vi "Example 1.vi"(8 "error in (no error)":errorcluster) -> (0 "error out":errorcluster)   [LabVIEW 2021, in "Named Timers.lvlib"]
uses:
  Named Timers.lvlib
  bc7bc3af-0b1d-4bbd-b21e-fb7784355964.vi
  7345f343-11d4-4018-b647-47a13be3ef10.vi
  f1f7e482-33cc-452b-8412-1830cebe123d.vi
panel:
  out "Number of timers":i32
  out "Timers":string[](array[string])
  in  "Use case":enum16{"Use case 1", "Use case 2", "Use case 3"}(ring)
  out "Timer 3 Elapsed time (ms)":u32
  out "Timer 2 Elapsed time (ms)":u32
  out "Timer 1 Elapsed time (ms)":u32
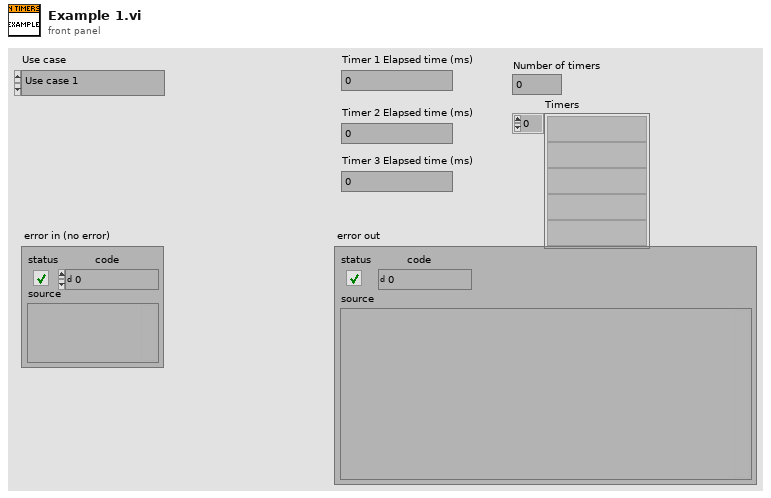
[diagram p1: front panel]
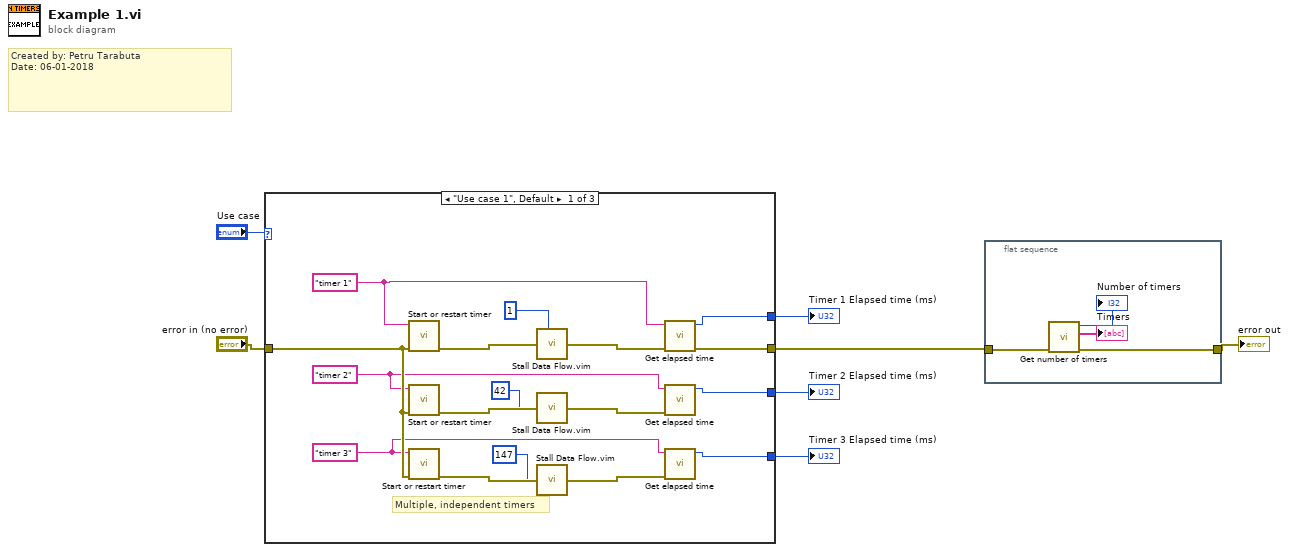
[diagram p0: block diagram]
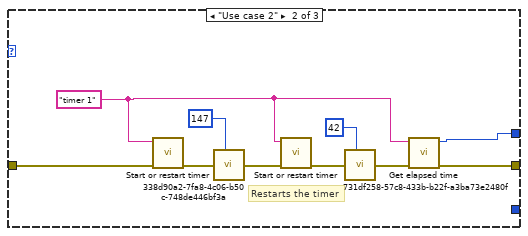
[diagram p2: hidden frame]
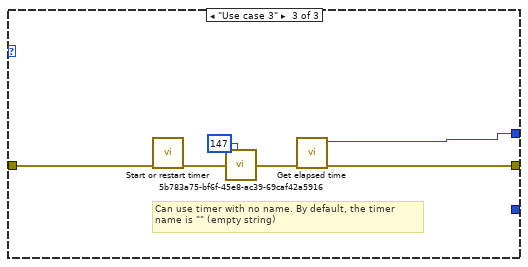
[diagram p3: hidden frame]
diagram:
  # "Created by: Petru Tarabuta\nDate: 06-01-2018"
  n1 = case shown="\"Use case 1\", Default" "Use case" {
    tunnel: [w24 w34 w40] -> w7
    tunnel: "error in (no error)" -> [w21 w31 w37]
    tunnel: [w10 _ _] -> w3
    tunnel: [w9 _ _] -> w2
    tunnel: [w8 w25 w35] -> w1
    frame "Use case 1", Default {
      w15 = "timer 3" ("Timer name")
      w19 = "timer 2" ("Timer name")
      w11 = "timer 1" ("Timer name")
      # "Multiple, independent timers"
      n2 = call "Start or restart timer.vi"("error in (no error)"=w21, "Timer name"=w11) -> ("error out"=w20:errorcluster)  [unwired: 9 in]
      n3 = call "Start or restart timer.vi"("error in (no error)"=w21, "Timer name"=w19) -> ("error out"=w18:errorcluster)  [unwired: 9 in]
      n4 = call "Start or restart timer.vi"("error in (no error)"=w21, "Timer name"=w15) -> ("error out"=w14:errorcluster)  [unwired: 9 in]
      n5 = call "Stall Data Flow.vim"("value in"=w20, "milliseconds to wait"=u32 1) -> ("value out"=w23:errorcluster)  [unwired: 1 out]
      n6 = call "Stall Data Flow.vim"("value in"=w18, "milliseconds to wait"=u32 42) -> ("value out"=w17:errorcluster)  [unwired: 1 out]
      n7 = call "Stall Data Flow.vim"("value in"=w14, "milliseconds to wait"=u32 147) -> ("value out"=w13:errorcluster)  [unwired: 1 out]
      n8 = call "Get elapsed time.vi"("error in (no error)"=w23, "Timer name"=w11) -> ("error out"=w24:errorcluster, "Elapsed time (ms)"=w8:u32)  [unwired: 6 in, 2 out]
      n9 = call "Get elapsed time.vi"("error in (no error)"=w17, "Timer name"=w19) -> ("Elapsed time (ms)"=w9:u32)  [unwired: 6 in, 3 out]
      n10 = call "Get elapsed time.vi"("error in (no error)"=w13, "Timer name"=w15) -> ("Elapsed time (ms)"=w10:u32)  [unwired: 6 in, 3 out]
    }
    frame "Use case 2" {
      w28 = "timer 1" ("Timer name")
      # "Restarts the timer"
      n11 = call "Start or restart timer.vi"("error in (no error)"=w31, "Timer name"=w28) -> ("error out"=w30:errorcluster)  [unwired: 9 in]
      n12 = call "338d90a2-7fa8-4c06-b50c-748de446bf3a.vi"("value in"=w30, "milliseconds to wait"=u32 147) -> ("value out"=w33:errorcluster)  [unwired: 1 out]
      n13 = call "Start or restart timer.vi"("error in (no error)"=w33, "Timer name"=w28) -> ("error out"=w29:errorcluster)  [unwired: 9 in]
      n14 = call "731df258-57c8-433b-b22f-a3ba73e2480f.vi"("value in"=w29, "milliseconds to wait"=u32 42) -> ("value out"=w27:errorcluster)  [unwired: 1 out]
      n15 = call "Get elapsed time.vi"("error in (no error)"=w27, "Timer name"=w28) -> ("error out"=w34:errorcluster, "Elapsed time (ms)"=w25:u32)  [unwired: 6 in, 2 out]
    }
    frame "Use case 3" {
      # "Can use timer with no name. By default, the timer name is \"\" (empty string)"
      n16 = call "Start or restart timer.vi"("error in (no error)"=w37) -> ("error out"=w36:errorcluster)  [unwired: 10 in]
      n17 = call "5b783a75-bf6f-45e8-ac39-69caf42a5916.vi"("value in"=w36, "milliseconds to wait"=u32 147) -> ("value out"=w39:errorcluster)  [unwired: 1 out]
      n18 = call "Get elapsed time.vi"("error in (no error)"=w39) -> ("error out"=w40:errorcluster, "Elapsed time (ms)"=w35:u32)  [unwired: 7 in, 2 out]
    }
  }
  "Timer 1 Elapsed time (ms)" <- w1
  "Timer 2 Elapsed time (ms)" <- w2
  "Timer 3 Elapsed time (ms)" <- w3
  n19 = flat-sequence {
    tunnel: w7 -> [w44]
    tunnel: [w43] -> w5
    frame #0 {
      n20 = call "Get number of timers.vi"("error in (no error)"=w44) -> ("error out"=w43:errorcluster, "Timers"=→"Timers":string[], "Number of timers"=→"Number of timers":i32)  [unwired: 8 in]
    }
  }
  "error out" <- w5
